vi "device extract module id from case id string.vi"(10 "dest_module_id":u32, 11 "case_id":string) -> (2 "dest_module_id out":u32, 3 "function return":i32)   [LabVIEW 2019, in "apdm.lvlib"]
doc: "APDM_EXPORT int apdm_device_extract_module_id_from_case_id_string(const char *case_id, uint32_t *dest_module_id);"
uses:
  apdm.lvlib
  Lee Lab/CP FES Walking 2018/Code/Working/LabVIEW/apdm.dll
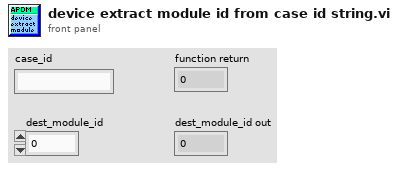
[diagram p1: front panel]
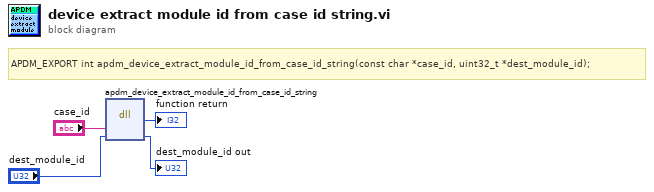
[diagram p0: block diagram]
diagram:
  # "APDM_EXPORT int apdm_device_extract_module_id_from_case_id_string(const char *case_id, uint32_t *dest_module_id);"
  n1 = dll-call lib="C:/Users/jfalesi/Dropbox/Lee Lab/CP FES Walking 2018/Code/Working/LabVIEW/apdm.*" fn="apdm_device_extract_module_id_from_case_id_string"("case_id"="case_id", "dest_module_id"="dest_module_id") -> (→"function return":i32, "dest_module_id"=→"dest_module_id out":u32)  [unwired: 4 in, 2 out]
